vi "Host-Version-Top-Level.vi"() -> ()   [LabVIEW 2015]
panel:
  in  "Run #\nto Load":i32=1
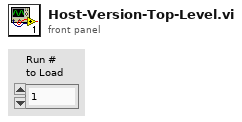
[diagram p1: front panel]
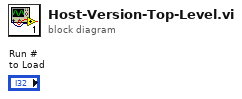
[diagram p0: block diagram]
diagram:
